vi "config_and_acquire_OSC.vi"() -> ()   [LabVIEW 2011]
doc: "Demonstrates how to set up an oscilloscope automatically. You can configure this VI to acquire a waveform from a single channel by following the following steps:\n\n1. Specify a valid VISA resource to use. \n2. Specify a channel. \n3. Specify a time-out value for reading a waveform.\n4. Run this VI. The <B>Waveform Graph</B> displays the waveform you acquire."
uses:
  <instrlib>/Tektronix 7000 Series/Tektronix 7000 Series.lvlib
  <instrlib>/Tektronix 7000 Series/Public/Configure/Configure Trigger (Edge).vi
  <instrlib>/Tektronix 7000 Series/Public/Data/Read (Single Waveform).vi
panel:
  in  "start":bool
  in  "Tab Control":enum32{"config", "measurement"}(tab)
  in  "Trigger":refnum<visa-resource-name>
  in  "OSC":refnum<visa-resource-name>
  in  "Trigger Channel":u16(ring)=1 items=["Channel1"=0, "Channel2"=1, "Channel3"=2, "Channel4"=3, "Aux"=12, "Line"=13, "Digital Channel0"=14, "Digital Channel1"=15, "Digital Channel2"=16, "Digital Channel3"=17, "Digital Channel4"=18, "Digital Chennel5"=19, "Digital Channel6"=20, "Digital Channel7"=21, "Digital Channel8"=22, "Digital Channel9"=23, "Digital Channel10"=24, "Digital Channel11"=25, "Digital Channel12"=26, "Digital Channel13"=27, "Digital Channel14"=28, "Digital Channel15"=29]
  in  "Trigger Level":dbl=3.0 format="%.1f"
  in  "Timebase":dbl=4.0
  in  "Record Length":u32=10000 caption="Record Length (10000s)" step=1
  in  "Acquisition Type":u16(ring) items=["Sample", "Peak Detect", "Hi Res", "Average", "Envelope", "WfmDB"]
  in  "Average#":i32=10
  in  "Envelope Waveforms":i32=10
  in  "Sampling Modes":T1(ring)=enum."Equivalent"
  out "Waveform Graph":waveform(dbl)(graph)
  in  "Meas Channel":u16(ring) items=["Channel 1", "Channel 2", "Channel 3", "Channel 4", "Math 1", "Math 2", "Math 3", "Math 4", "Reference 1", "Reference 2", "Reference 3", "Reference 4"]
  in  "Maximum Time":u32=10000
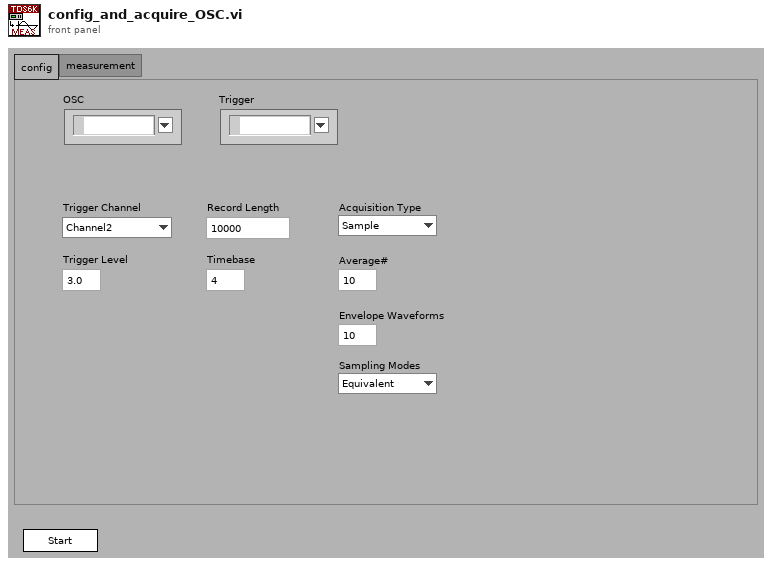
[diagram p1: front panel]
types:
  T1 = enum16{"Real Time", "Interpolater", "Equivalent"}
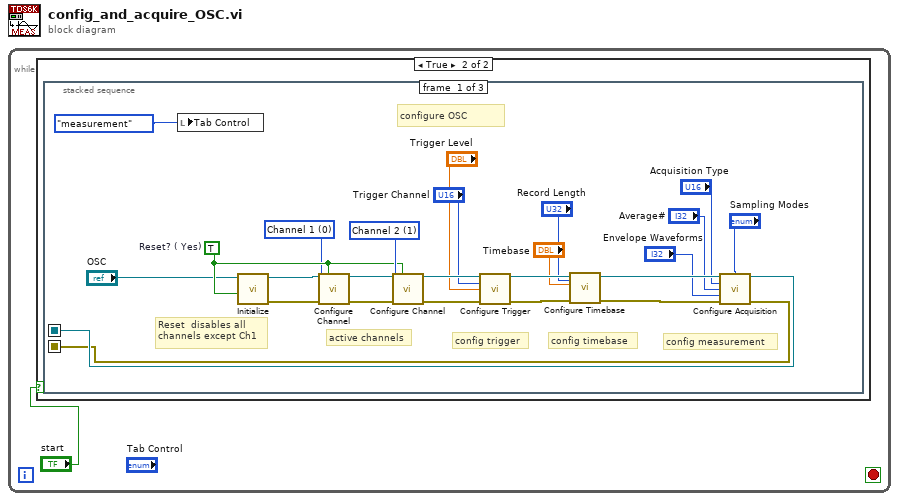
[diagram p0: block diagram]
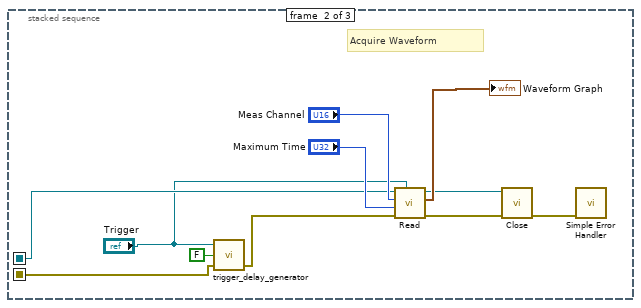
[diagram p3: hidden frame]
diagram:
  n1 = while {
    stop <- _ stop-if-true
    n2 = case shown="True" "start" {
      frame False {
      }
      frame True {
        n3 = stacked-sequence {
          seq-local: [w5 _ _] -> [_ w35 _]
          seq-local: [w4 _ _] -> [_ w29 _]
          frame #0 {
            w10 = u16 1 items=["Channel 1", "Channel 2", "Channel 3", "Channel 4", "Math 1", "Math 2", "Math 3", "Math 4", "Reference 1", "Reference 2", "Reference 3", "Reference 4"] ("Channel (0: Channel 1)")
            w8 = u16 0 items=["Channel 1", "Channel 2", "Channel 3", "Channel 4", "Math 1", "Math 2", "Math 3", "Math 4", "Reference 1", "Reference 2", "Reference 3", "Reference 4"] ("Channel (0: Channel 1)")
            w9 = TRUE  # Reset? ( Yes)
            # "config measurement"
            # "config timebase"
            # "configure OSC"
            # "active channels"
            # "config trigger"
            # "Reset  disables all \nchannels except Ch1"
            n4 = local write "Tab Control"(enum32{"config", "measurement"}."measurement" ("Tab Control")) -> ()
            n5 = call <instrlib>:"Initialize.vi"("Reset? ( Yes)"=w9, "VISA resource name"="OSC") -> ("error out"=w19:errorcluster, "VISA resource name out"=w15:refnum<visa-resource-name>)  [unwired: 8 in]
            n6 = call <instrlib>:"Configure Channel.vi"("VISA resource name"=w15, "Enable Channel (T: Enable)"=w9, "Channel (0: Channel 1)"=w8, "error in (no error)"=w19) -> ("VISA resource name out"=w16:refnum<visa-resource-name>, "error out"=w20:errorcluster)  [unwired: 10 in]
            n7 = call <instrlib>:"Configure Channel.vi"("VISA resource name"=w16, "Enable Channel (T: Enable)"=w9, "Channel (0: Channel 1)"=w10, "error in (no error)"=w20) -> ("VISA resource name out"=w17:refnum<visa-resource-name>, "error out"=w21:errorcluster)  [unwired: 10 in]
            n8 = call-poly <instrlib>:"Configure Trigger.vi"("VISA resource name"=w17, "Source (0:Channel1)"="Trigger Channel", "Trigger Level (0.0V)"="Trigger Level", "error in (no error)"=w21) -> ("VISA resource name out"=w18:refnum<visa-resource-name>, "error out"=w22:errorcluster)  [unwired: 10 in]
            n9 = call <instrlib>:"Configure Timebase.vi"("Record Length (10000)"="Record Length", "error in (no error)"=w22, "Timebase (4 ns)"="Timebase", "VISA resource name"=w18) -> ("error out"=w26:errorcluster, "VISA resource name out"=w25:refnum<visa-resource-name>)  [unwired: 6 in]
            n10 = call <instrlib>:"Configure Acquisition.vi"("VISA resource name"=w25, "Acquisition Type (0:Sample)"="Acquisition Type", "Average Waveforms (10)"="Average#", "Envelope Waveforms (10)"="Envelope Waveforms", "error in (no error)"=w26, "Sampling Modes (Real Time)"="Sampling Modes") -> ("VISA resource name out"=w5:refnum<visa-resource-name>, "error out"=w4:errorcluster)  [unwired: 8 in]
          }
          frame #1 {
            # "Acquire Waveform"
            n11 = call "trigger_delay_generator.vi"("error in (no error)"=w29, "Boolean"=FALSE, "VISA resource name"="Trigger") -> ("error out"=w28:errorcluster)  [unwired: 1 in, 1 out]
            n12 = call-poly <instrlib>:"Read.vi"("Trigger"="Trigger", "error in (no error)"=w28, "Maximum Time (10000 ms)"="Maximum Time", "Channel (0: Channel 1)"="Meas Channel", "VISA resource name"=w35) -> ("error out"=w31:errorcluster, "Waveform Data"=→"Waveform Graph":waveform(dbl), "VISA resource name out"=w32:refnum<visa-resource-name>)  [unwired: 4 in]
            n13 = call <instrlib>:"Close.vi"("error in (no error)"=w31, "VISA resource name"=w32) -> ("error out"=w33:errorcluster)  [unwired: 9 in]
            n14 = call <vilib>:"Simple Error Handler.vi"("error in (no error)"=w33) -> ()  [unwired: 4 in, 5 out]
          }
          frame #2 {
            # "close connection and look for errors"
          }
        }
      }
    }
  }
